vi "ToggleArmingSystem.vi"(0 "reference in":refnum<class "SecuritySystem.lvclass">, 5 "Error In":errorcluster) -> (14 "reference out":refnum<class "SecuritySystem.lvclass">, 19 "Error Out":errorcluster)   [LabVIEW 2024, in "SecuritySystem.lvclass"]
uses:
  SecuritySystem.lvclass
  SecuritySystem.lvclass/SecuritySystem.ctl
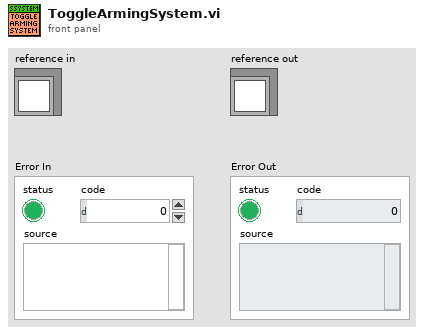
[diagram p1: front panel]
types:
  T1 = typedef "SecuritySystem.lvclass/ObjectAttributes.ctl" = cluster{"Rooms":map{variant, variant}}
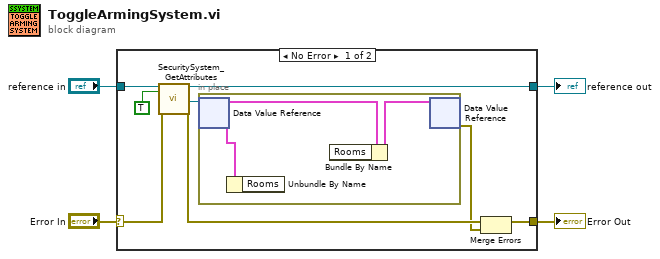
[diagram p0: block diagram]
diagram:
  n1 = case shown="No Error" "Error In" {
    selector: "Error In" -> [w11 w16]
    tunnel: [w9 w16] -> w3
    tunnel: [w10 w15] -> w1
    tunnel: "reference in" -> [w12 w15]
    frame No Error {
      n2 = call "SecuritySystem_GetAttributes.vi"("reference in"=w12, "OnlyGetDvrReference(False)"=TRUE, "Error In"=w11) -> ("reference out"=w10:refnum<class "SecuritySystem.lvclass">, "DataRef"=w8:refnum<data-value>, "Error Out"=w6:errorcluster)  [unwired: 13 in, 1 out]
      n3 = in-place {
        n4 = in-place-dvr #1(w8) -> (w13:T1)  [unwired: 1 out]
        n5 = Unbundle By Name(w13) -> ()  [unwired: 1 out]
        n6 = Bundle By Name(cluster=w13) -> (w14:T1)  [unwired: 1 in]
        n7 = in-place-dvr #1(w14) -> (w5:errorcluster)  [unwired: 1 out]
      }
      n8 = Merge Errors(w6, w5) -> (w9:errorcluster)
    }
    frame Error {
    }
  }
  "Error Out" <- w3
  "reference out" <- w1
